vi "Pad Version Number.vi"(1 "Desired minimum number of fields (Dflt = 4)":i32=4, 2 "Input Version Number":string) -> (0 "Output Version Number (padded)":string)   [LabVIEW 2023, in "Error Manager.lvlib"]
doc: "This VI pads (extends) a version number such as \"1.0\" to a version number such as \"1.0.0.0\"."
uses:
  Error Manager.lvlib
panel:
  out "T = Need to pad":bool
  out "Number of fields of input":i32
  # "Input\nInputs to the VI"
  # "Development\nControls or indicators that are useful for development or testing, but which are not outputs of the VI."
  # "Output\nOutputs of the VI"
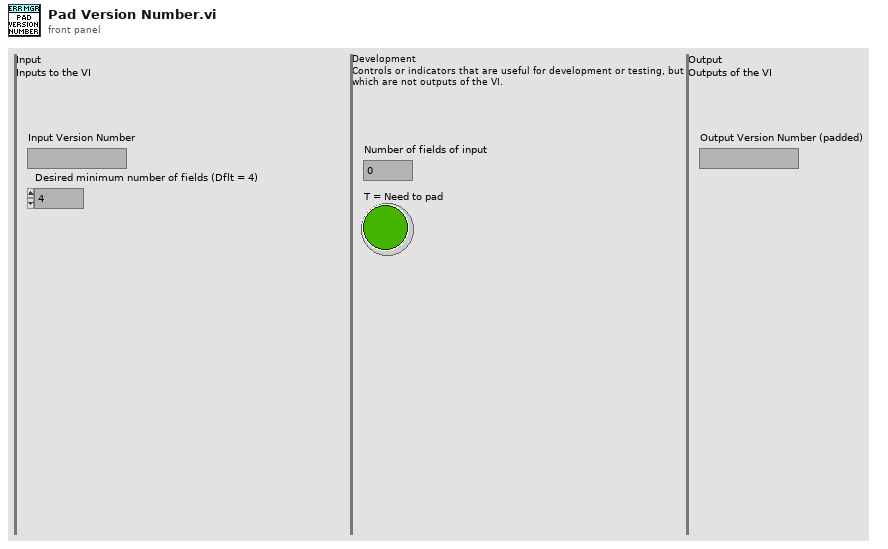
[diagram p1: front panel]
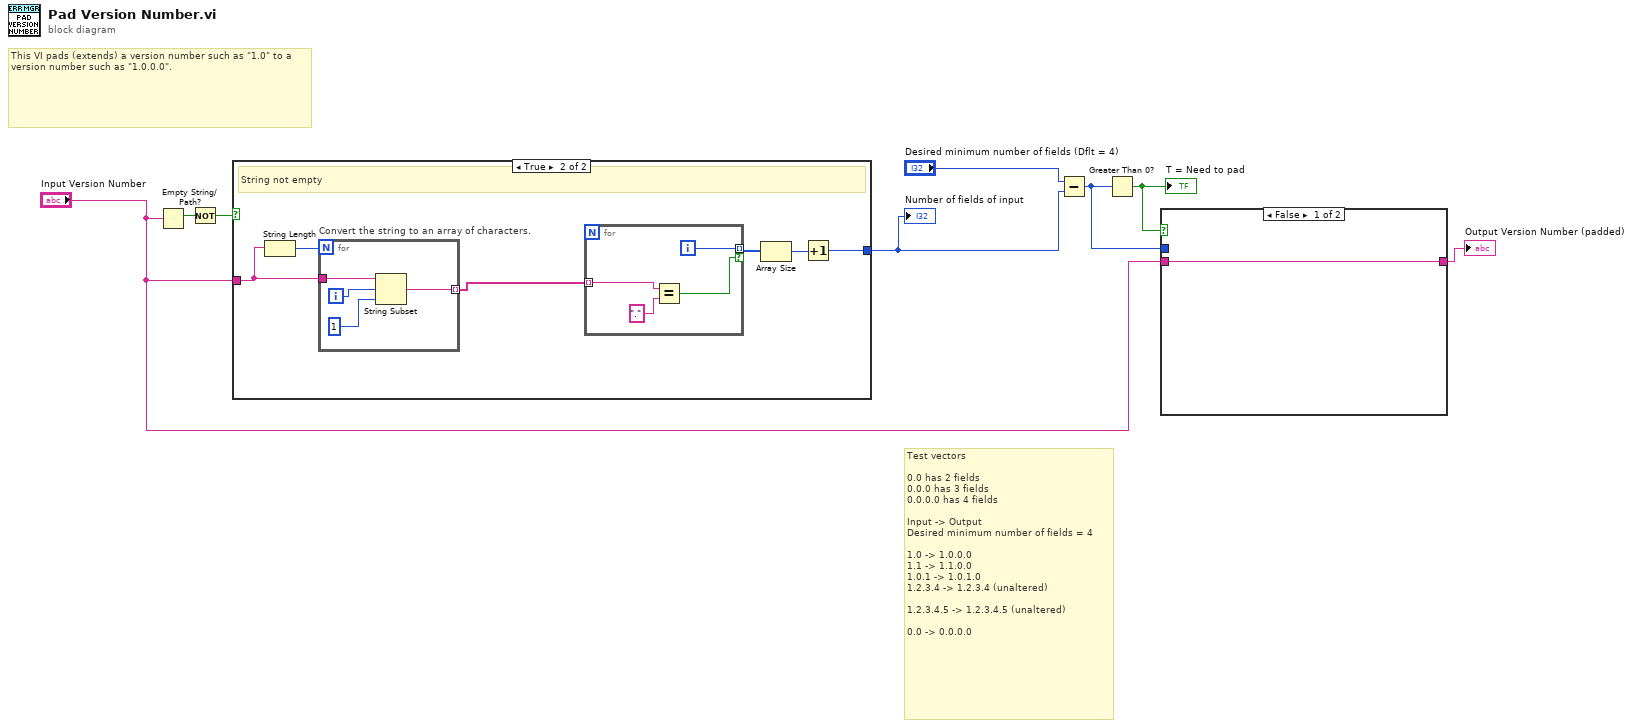
[diagram p0: block diagram]
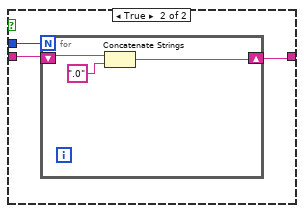
[diagram p2: hidden frame]
diagram:
  # "This VI pads (extends) a version number such as \"1.0\" to a version number such as \"1.0.0.0\"."
  # "Test vectors\n\n0.0 has 2 fields\n0.0.0 has 3 fields\n0.0.0.0 has 4 fields\n\nInput -> Output\nDesired minimum number of fields = 4\n\n1.0 -> 1.0.0.0\n1.1 -> 1.1.0.0\n1.0.1 -> 1.0.1.0\n1.2.3.4 -> 1.2.3.4 (unaltered)\n\n1.2.3.4.5 -> 1.2.3.4.5 (unaltered)\n\n0.0 -> 0.0.0.0"
  n1 = Empty String/Path?(string/path="Input Version Number") -> (empty?=w8:bool)
  n2 = Not(x=w8) -> (.not. x?=w7:bool)
  n3 = case shown="True" w7 {
    tunnel: "Input Version Number" -> [_ w10]
    tunnel: [_ w12] -> w5
    frame False {
    }
    frame True {
      # "String not empty"
      n4 = String Length(string=w10) -> (length=w11:i32)
      n5 = for "Convert the string to an array of characters." {
        N: w11 -> [_]
        tunnel: w10 -> [w16]
        tunnel: [w17] -> w9 mode=indexing
        i -> [w15]
        n6 = String Subset(string=w16, offset (0)=w15, length (rest)=1 ("length (rest)")) -> (substring=w17:string)
      }
      n7 = for {
        tunnel: w9 -> [w22] mode=indexing
        tunnel: [w20] -> w14 mode=indexing if=w19
        i -> [w20]
        n8 = Equal?(x=w22, y=".") -> (x = y?=w19:bool)
      }
      n9 = Array Size(array=w14) -> (size(s)=w13:i32)
      n10 = Increment(x=w13) -> (x+1=w12:i32)
    }
  }
  "Number of fields of input" <- w5
  n11 = Subtract(x="Desired minimum number of fields (Dflt = 4)", y=w5) -> (x-y=w4:i32)
  n12 = Greater Than 0?(x=w4) -> (x > 0?=w3:bool)
  "T = Need to pad" <- w3
  n13 = case shown="False" w3 {
    tunnel: w4 -> [_ w26]
    tunnel: "Input Version Number" -> [w23 w25]
    tunnel: [w23 w24] -> w1
    frame False {
    }
    frame True {
      n14 = for {
        N: w26 -> [_]
        shift-right: [w27] -> w24
        shift-left: w25 -> [w29]
        n15 = Concatenate Strings(w29, ".0") -> (w27:string)
      }
    }
  }
  "Output Version Number (padded)" <- w1
